vi "FGEN Self-Test.vi"(8 "error in (no error)":errorcluster, 11 "Function Generator in":refnum<class "Function Generator.lvclass">) -> (0 "error out":errorcluster, 2 "Report Text":string, 3 "Function Generator out":refnum<class "Function Generator.lvclass">)   [LabVIEW 2023, in "HardwareAbstractionLayer_LVOOP.lvlib" / "Function Generator.lvclass"]
uses:
  Function Generator.lvclass
  Function Generator.lvclass/Function Generator.ctl
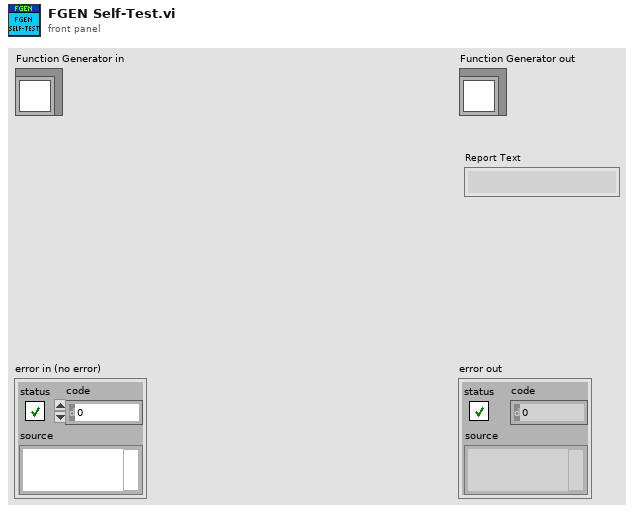
[diagram p1: front panel]
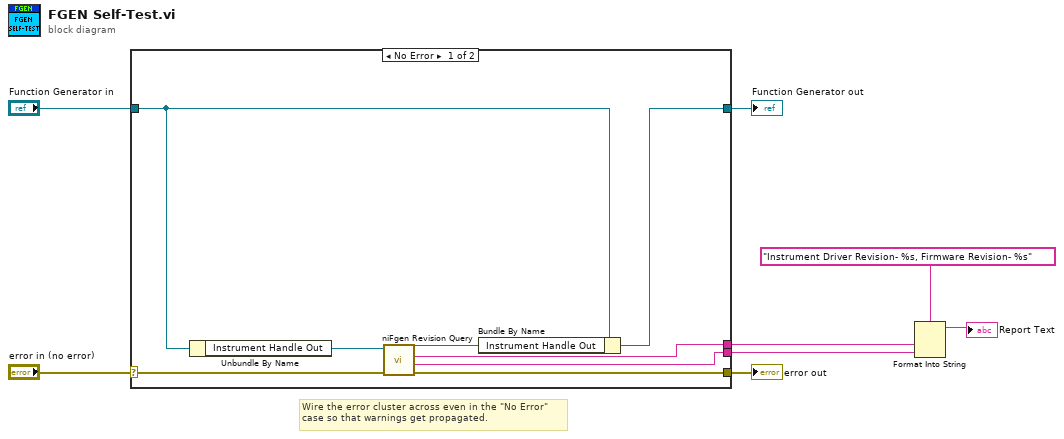
[diagram p0: block diagram]
diagram:
  # "Wire the error cluster across even in the \"No Error\"\ncase so that warnings get propagated."
  n1 = case shown="No Error" "error in (no error)" {
    selector: "error in (no error)" -> [w15 w18]
    tunnel: [w14 w18] -> w7
    tunnel: [w12 w17] -> w5
    tunnel: "Function Generator in" -> [w13 w17]
    tunnel: [w10 _] -> w2
    tunnel: [w9 _] -> w1
    frame No Error {
      n2 = Unbundle By Name(w13) -> ("Instrument Handle Out"=w16:refnum<k15>)
      n3 = call <instrlib>:"niFgen Revision Query.vi"("error in (no error)"=w15, "Instrument Handle"=w16) -> ("error out"=w14:errorcluster, "Firmware Revision"=w9:string, "Instrument Driver Revision"=w10:string, "Instrument Handle Out"=w11:refnum<k15>)  [unwired: 6 in]
      n4 = Bundle By Name(cluster=w13, "Instrument Handle Out"=w11) -> (w12:refnum<class "Function Generator.lvclass">)
    }
    frame Error {
    }
  }
  "error out" <- w7
  "Function Generator out" <- w5
  n5 = Format Into String(format string="Instrument Driver Revision- %s, Firmware Revision- %s", w2, w1) -> (resulting string=→"Report Text":string)  [unwired: 2 in, 1 out]
